vi "Begin.vi"   [LabVIEW 2019]
uses:
  <vilib>/Rock Robotics/SystemInterfaces/AI/FPGA_AIChannel.ctl
  frc-software-2019/Transducer.ctl
types:
  T1 = typedef "Transducer.ctl" = enum16{"Transducer"}
  T2 = typedef "FPGA_AIChannel.ctl" = enum8{"AI 0", "AI 1", "AI 2", "AI 3", "AI MXP 0", "AI MXP 1", "AI MXP 2", "AI MXP 3", "Invalid"}
  T3 = typedef "WPI_AnalogChannelDevRef.ctl" = cluster{"DevStatus":errorcluster, "Analog Channel":T2}
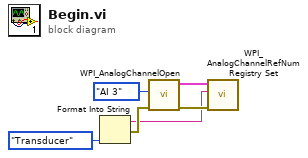
[diagram p0: block diagram]
diagram:
  n1 = Format Into String(Transducer."Transducer") -> (resulting string=w3:string, error out=w6:errorcluster)  [unwired: 3 in]
  n2 = call <vilib>:"WPI_AnalogChannelOpen.vi"("error in (no error)"=w6, "Analog Channel"=FPGA_AIChannel."AI 3") -> ("error out"=w5:errorcluster, "AIDeviceRef"=w4:T3)  [unwired: 8 in]
  n3 = call <vilib>:"WPI_AnalogChannelRefNum Registry Set.vi"("error in (no error)"=w5, "refnum name"=w3, "AIDeviceRef"=w4) -> ()  [unwired: 7 in, 2 out]
